vi "CreateSlide.vi"(8 "error in (no error)":errorcluster, 9 "Type (FP)":T1=enum."FP", 10 "Path":path) -> (0 "error out":errorcluster, 3 "BD Slide":refnum<class "Slide.lvclass">)   [LabVIEW 2017, in "Slide.lvclass"]
uses:
  Slide.lvclass
  SlideType.ctl
  Slide.lvclass/Slide.ctl
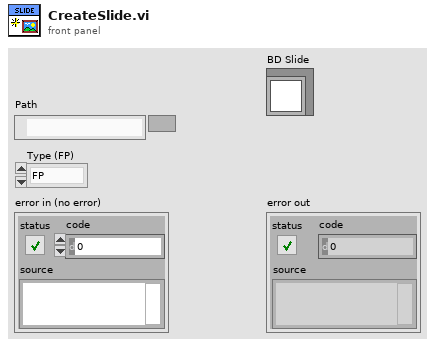
[diagram p1: front panel]
types:
  T1 = typedef "Slide.lvclass/SlideType.ctl" = enum16{"Image", "FP", "BD", "VI-Run"}
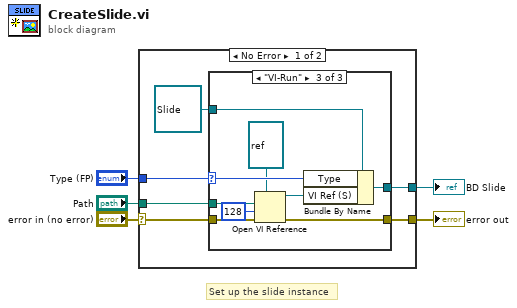
[diagram p0: block diagram]
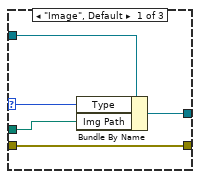
[diagram p2: hidden frame]
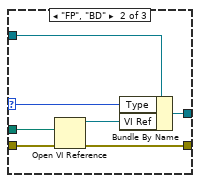
[diagram p3: hidden frame]
diagram:
  # "Set up the slide instance"
  n1 = case shown="No Error" "error in (no error)" {
    selector: "error in (no error)" -> [w7 w33]
    tunnel: [w6 w33] -> w4
    tunnel: [w10 _] -> w3
    tunnel: "Type (FP)" -> [w9 _]
    tunnel: "Path" -> [w8 _]
    frame No Error {
      n2 = case shown="\"VI-Run\"" w9 {
        selector: w9 -> [w14 w20 w29]
        tunnel: refnum<class "Slide.lvclass"> refnum ("Slide.lvclass") -> [w15 w22 w31]
        tunnel: [w16 w21 w30] -> w10
        tunnel: w8 -> [w13 w19 w28]
        tunnel: w7 -> [w12 w18 w27]
        tunnel: [w12 w17 w26] -> w6
        frame "Image", Default {
          n3 = Bundle By Name(cluster=w15, "Type"=w14, "Img Path"=w13) -> (w16:refnum<class "Slide.lvclass">)
        }
        frame "FP", "BD" {
          n4 = Open VI Reference(vi path=w19, error in (no error)=w18) -> (vi reference=w23:refnum<vi>, error out=w17:errorcluster)  [unwired: 4 in]
          n5 = Bundle By Name(cluster=w22, "Type"=w20, "VI Ref"=w23) -> (w21:refnum<class "Slide.lvclass">)
        }
        frame "VI-Run" {
          n6 = Open VI Reference(type specifier VI Refnum (for type only)=refnum<vi> refnum, vi path=w28, options=128, error in (no error)=w27) -> (vi reference=w32:refnum<vi>, error out=w26:errorcluster)  [unwired: 2 in]
          n7 = Bundle By Name(cluster=w31, "Type"=w29, "VI Ref (S)"=w32) -> (w30:refnum<class "Slide.lvclass">)
        }
      }
    }
    frame Error {
    }
  }
  "BD Slide" <- w3
  "error out" <- w4
